vi "To PV Data.vi"(8 "error in":errorcluster, 10 "PV data in":refnum<class "PV Data.lvclass">, 11 "Base Interface in":refnum<class "Base Interface.lvclass">) -> (0 "error out":errorcluster, 2 "PV data out":refnum<class "PV Data.lvclass">, 3 "Base Interface out":refnum<class "Base Interface.lvclass">)   [LabVIEW 2020, in "PV Access.lvlib" / "PV Data.lvlib" / "Base Interface.lvclass"]
uses:
  Base Interface.lvclass
  PV Data/PV Data.lvclass
  PV Data/Write Field - Variant.vi
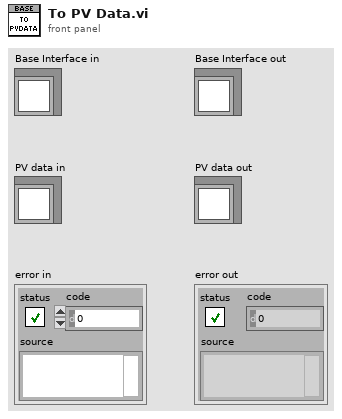
[diagram p1: front panel]
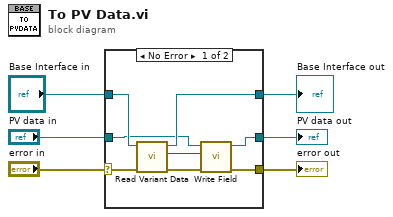
[diagram p0: block diagram]
diagram:
  n1 = case shown="No Error" "error in" {
    selector: "error in" -> [w10 w17]
    tunnel: [w12 w17] -> w3
    tunnel: [w14 w16] -> w1
    tunnel: "Base Interface in" -> [w13 w16]
    tunnel: "PV data in" -> [w9 w15]
    tunnel: [w8 w15] -> w2
    frame No Error {
      n2 = call-dynamic "Read Variant Data.vi"("error in"=w10, "Base Interface in"=w13) -> ("error out"=w11:errorcluster, "data"=w7:variant, "Base Interface out"=w14:refnum<class "Base Interface.lvclass">)  [unwired: 7 in]
      n3 = call-poly "Write Field.vi"("error in (no error)"=w11, "value in"=w7, "PV Data in"=w9) -> ("error out"=w12:errorcluster, "PV Data out"=w8:refnum<class "PV Data.lvclass">)  [unwired: 6 in, 1 out]
    }
    frame Error {
    }
  }
  "error out" <- w3
  "Base Interface out" <- w1
  "PV data out" <- w2
